vi "citTemplate.VariantToEnumDescriptor.vi"(7 "Variant enum data":variant) -> (8 "enum type descriptor":string)   [LabVIEW 2016]
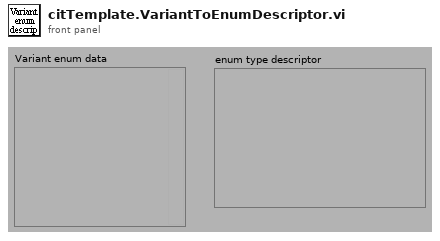
[diagram p1: front panel]
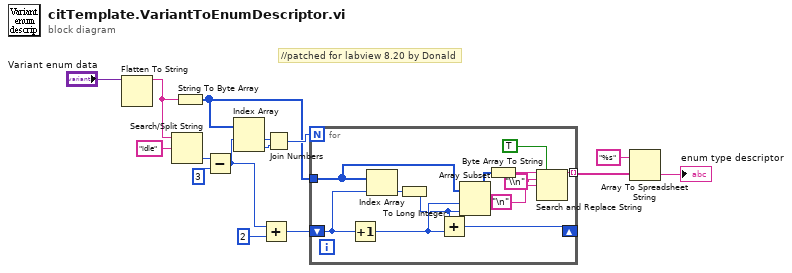
[diagram p0: block diagram]
diagram:
  # "//patched for labview 8.20 by Donald"
  n1 = Flatten To String(anything="Variant enum data") -> (data string=w9:string)  [unwired: 1 in, 4 out]
  n2 = Search/Split String(string=w9, search string/char (-)="idle") -> (offset of match=w10:i32)  [unwired: 3 out]
  n3 = String To Byte Array(string=w9) -> (unsigned byte array=w5:u8[])
  n4 = Subtract(x=w10, y=3) -> (x-y=w4:i32)
  n5 = Index Array(array=w5, index #1=w4) -> (element #1=w8:u8, element #2=w7:u8)  [unwired: 1 in]
  n6 = Add(x=w4, y=2) -> (x+y=w2:i32)
  n7 = Join Numbers(hi=w8, lo=w7) -> ((hi.lo)=w6:u16)
  n8 = for {
    N: w6 -> [_]
    tunnel: w5 -> [w27]
    shift-right: [w25] -> _
    shift-left: w2 -> [w26]
    tunnel: [w17] -> w1 mode=indexing
    n9 = Increment(x=w26) -> (x+1=w24:i32)
    n10 = Index Array(array=w27, index=w26) -> (element=w23:u8)
    n11 = To Long Integer(number=w23) -> (32bit integer=w16:i32)
    n12 = Add(x=w16, y=w24) -> (x+y=w25:i32)
    n13 = Array Subset(array=w27, index=w24, length=w16) -> (w18:u8[])
    n14 = Byte Array To String(unsigned byte array=w18) -> (string=w22:string)
    n15 = Search and Replace String(replace all?=TRUE ("replace all? (F)"), input string=w22, search string="\\n", replace string="\n") -> (result string=w17:string)  [unwired: 1 in, 6 out]
  }
  n16 = Array To Spreadsheet String(array=w1, 3:"%s" ("format string")) -> (spreadsheet string=→"enum type descriptor":string)  [unwired: 1 out]
